vi "S30c_dll F32.vi"(4 "error in":errorcluster, 6 "Nr.":u8, 7 "Dev Addr":u8=250) -> (0 "error out":errorcluster, 2 "Config Byte":u8)   [LabVIEW 2014, in "K_S30c_dll.lvlib"]
uses:
  K_S30c_dll.lvlib
  s30c.dll
panel:
  # "Function 32: Read configuration\n\nusing s30c.dll\nKeller AG für Druckmesstechnik, 29.5.08 b.v."
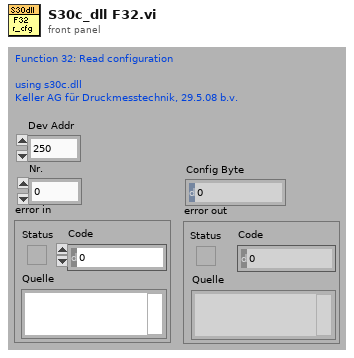
[diagram p1: front panel]
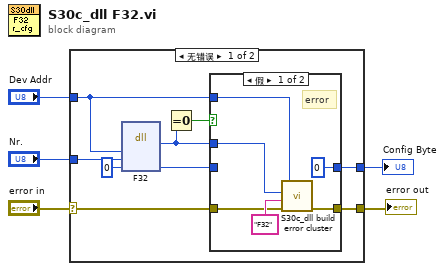
[diagram p0: block diagram]
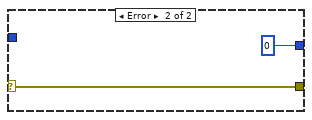
[diagram p3: hidden frame]
diagram:
  n1 = case shown="无错误" "error in" {
    selector: "error in" -> [w8 w23]
    tunnel: [w13 w23] -> w2
    tunnel: "Dev Addr" -> [w9 _]
    tunnel: "Nr." -> [w10 _]
    tunnel: [w6 u8 0 ("Coeff")] -> w3
    frame No Error {
      n2 = dll-call lib="PTH2Labs EworkSINOPEC北控自动相渗software2.08.5_dlls30c.dll" fn="F32"("DevAddr"=w9, "Coeff No"=w10, "Coeff"=u8 0) -> (w11:i16, "Coeff"=w7:u8)  [unwired: 5 in, 2 out]
      n3 = Equal To 0?(x=w11) -> (x = 0?=w14:bool)
      n4 = case shown="假" w14 {
        tunnel: [w20 w21] -> w13
        tunnel: w11 -> [w18 _]
        tunnel: w9 -> [w19 _]
        tunnel: w8 -> [w16 w21]
        tunnel: w7 -> [_ w22]
        tunnel: [u8 0 ("Coeff") w22] -> w6
        frame False {
          # "error"
          n5 = call "S30c_dll build error cluster.vi"("error in"=w16, "error Text"="F32", "error code"=w18, "Dev Addr"=w19) -> ("error out"=w20:errorcluster)  [unwired: 3 in]
        }
        frame True {
        }
      }
    }
    frame Error {
    }
  }
  "error out" <- w2
  "Config Byte" <- w3
